vi "Execute Step.vi"(8 "error in (no error)":errorcluster, 9 "result allocation in":T1, 10 "parameters":T1, 11 "Sequencer Module runtime in":refnum<class "Sequencer Module runtime.lvclass">) -> (0 "error out":errorcluster, 1 "results":T1, 2 "parameter allocation":T1, 3 "Sequencer Module runtime out":refnum<class "Sequencer Module runtime.lvclass">)   [LabVIEW 2015, in "Sequencer Module runtime.lvclass"]
uses:
  Sequencer Module runtime.lvclass
  <vilib>/NI/Tag Bus/table/data table.ctl
  Sequencer Module runtime.lvclass/Sequencer Module runtime.ctl
  classes/Sequence/Execution/Sequence.lvclass
  classes/Step/Execution/Step.lvclass
  <vilib>/NI/Tag Bus/table/data table.lvlib
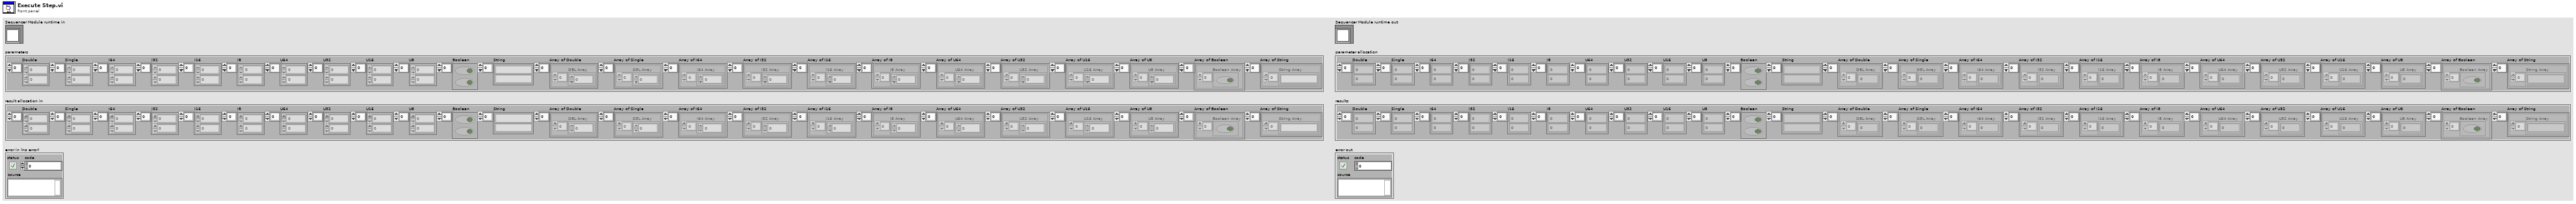
[diagram p1: front panel]
types:
  T1 = typedef "tag bus.lvlib/data table.lvlib/data table.ctl" = cluster{"Double":dbl[], "Single":sgl[], "I64":i64[], "I32":i32[], "I16":i16[], "I8":i8[], "U64":u64[], "U32":u32[], "U16":u16[], "U8":u8[], "Boolean":bool[], "String":string[], "Array of Double":cluster{"DBL Array":dbl[]}[], "Array of Single":cluster{"SGL Array":sgl[]}[], "Array of I64":cluster{"I64 Array":i64[]}[], "Array of I32":cluster{"I32 Array":i32[]}[], "Array of I16":cluster{"I16 Array":i16[]}[], "Array of I8":cluster{"I8 Array":i8[]}[], "Array of U64":cluster{"U64 Array":u64[]}[], "Array of U32":cluster{"U32 Array":u32[]}[], "Array of U16":cluster{"U16 Array":u16[]}[], "Array of U8":cluster{"U8 Array":u8[]}[], "Array of Boolean":cluster{"Boolean Array":bool[]}[], "Array of String":cluster{"String Array":string[]}[]}
  T2 = typedef "Step.lvclass/StepState.ctl" = cluster{"Step State":T3, "Flow Control":T4, "Jump Index":i32, "Done":bool}
  T3 = typedef "Step.lvclass/Step Status.ctl" = enum16{"Start", "Passed", "Failed", "Error", "Done", "Terminated", "Skipped", "Running"}
  T4 = typedef "Step.lvclass/Step Flow Control.ctl" = enum16{"Next Step", "Jump"}
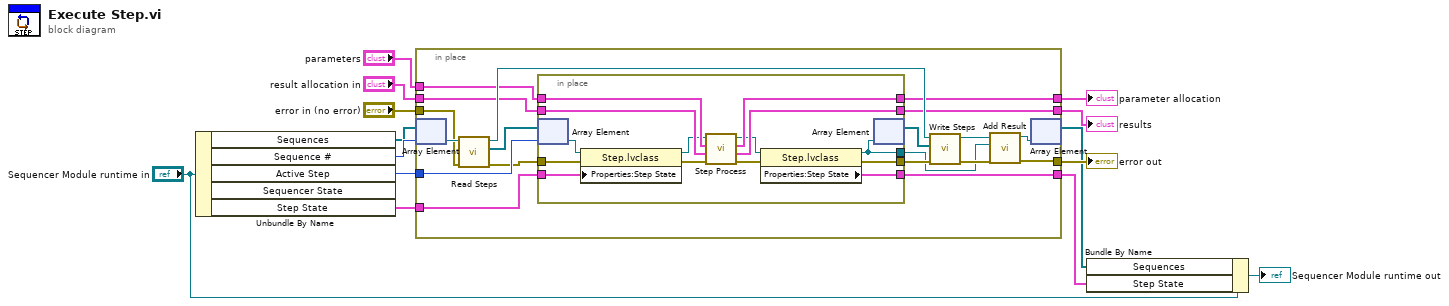
[diagram p0: block diagram]
diagram:
  n1 = Unbundle By Name("Sequencer Module runtime in") -> ("Sequences"=w9:refnum<class "Sequence.lvclass">[], "Sequence #"=w10:i32, "Active Step"=w11:i32, "Step State"=w12:T2)  [unwired: 1 out]
  n2 = in-place {
    in-place-border: w11 -> [w33]
    in-place-border: "error in (no error)" -> [w28]
    in-place-border: [w16] -> w14
    in-place-border: [w25] -> w7
    in-place-border: w12 -> [w24]
    in-place-border: "parameters" -> [w23]
    in-place-border: [w22] -> w4
    in-place-border: "result allocation in" -> [w21]
    in-place-border: [w20] -> w6
    n3 = in-place-array #1(w9, w10) -> (w32:refnum<class "Sequence.lvclass">)
    n4 = call-dynamic "Read Steps.vi"("error in (no error)"=w28, "Sequence in"=w32) -> ("error out"=w27:errorcluster, "Steps"=w31:refnum<class "Step.lvclass">[], "Sequence out"=w29:refnum<class "Sequence.lvclass">)  [unwired: 7 in]
    n5 = in-place {
      in-place-border: w27 -> [w40]
      in-place-border: [w35] -> w26
      in-place-border: [w37] -> w25
      in-place-border: w24 -> [w43]
      in-place-border: w23 -> [w47]
      in-place-border: [w46] -> w22
      in-place-border: w21 -> [w45]
      in-place-border: [w44] -> w20
      in-place-border: [w34] -> w15
      n6 = in-place-array #2(w31, w33) -> (w42:refnum<class "Step.lvclass">)
      n7 = property class="Step.lvclass"(reference=w42, error in=w40, "Properties:Step State"=w43) -> (reference out=w41:refnum<class "Step.lvclass">, error out=w39:errorcluster)
      n8 = call-dynamic "Step Process.vi"("error in (no error)"=w39, "result allocation"=w45, "parameters"=w47, "Step in"=w41) -> ("error out"=w36:errorcluster, "results"=w44:T1, "parameter allocation"=w46:T1, "Step out"=w38:refnum<class "Step.lvclass">)  [unwired: 4 in]
      n9 = property class="Step.lvclass"(reference=w38, error in=w36) -> (reference out=w34:refnum<class "Step.lvclass">, error out=w35:errorcluster, "Properties:Step State"=w37:T2)
      n10 = in-place-array #2(w34) -> (w30:refnum<class "Step.lvclass">[])  [unwired: 1 out]
    }
    n11 = call-dynamic "Write Steps.vi"("error in (no error)"=w26, "Steps"=w30, "Sequence in"=w29) -> ("error out"=w17:errorcluster, "Sequence out"=w19:refnum<class "Sequence.lvclass">)  [unwired: 7 in]
    n12 = call-dynamic "Add Result.vi"("error in (no error)"=w17, "Step"=w15, "Sequence in"=w19) -> ("error out"=w16:errorcluster, "Sequence out"=w18:refnum<class "Sequence.lvclass">)  [unwired: 7 in]
    n13 = in-place-array #1(w18) -> (w2:refnum<class "Sequence.lvclass">[])  [unwired: 1 out]
  }
  "error out" <- w14
  "results" <- w6
  "parameter allocation" <- w4
  n14 = Bundle By Name(cluster="Sequencer Module runtime in", "Sequences"=w2, "Step State"=w7) -> (→"Sequencer Module runtime out":refnum<class "Sequencer Module runtime.lvclass">)
